vi "Do Failure Action.vi"(7 "Assert Data":T1, 8 "error in (no error)":errorcluster, 11 "Failure Action in":refnum<class "Failure Action.lvclass">) -> (0 "error out":errorcluster)   [LabVIEW 2016, in "AssertEngine.lvlib" / "Failure Action.lvclass"]
uses:
  Failure Action.lvclass
  Log Assert/Assert Data.ctl
  AssertEngine.lvlib
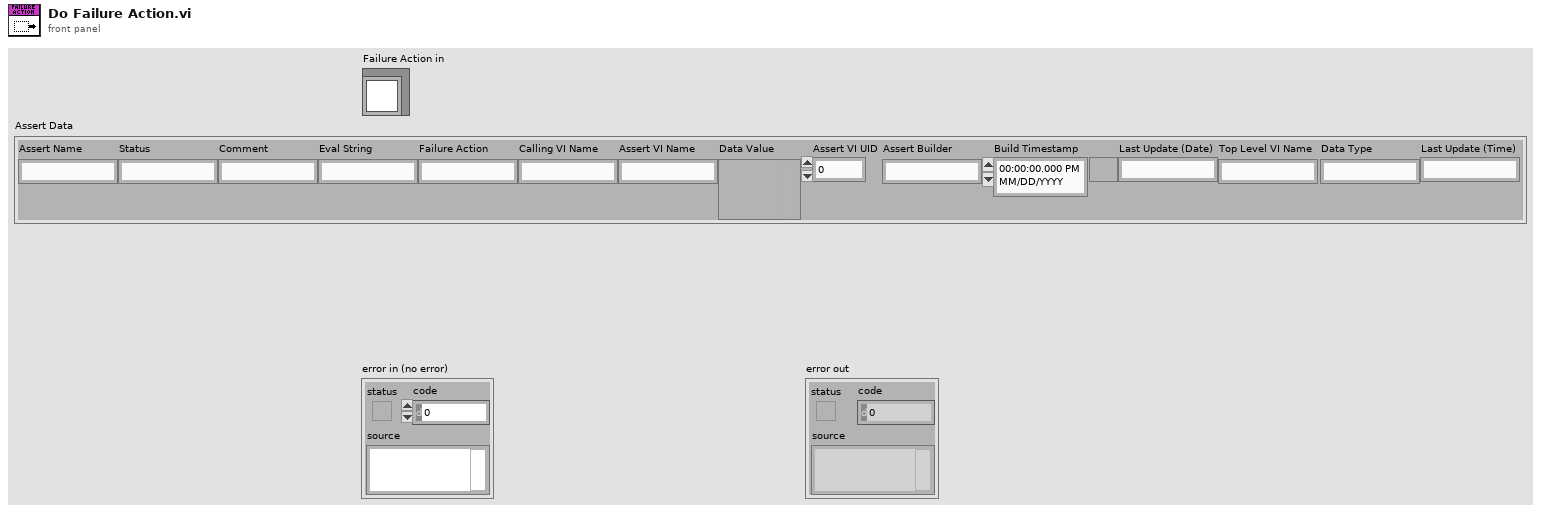
[diagram p1: front panel]
types:
  T1 = typedef "AssertEngine.lvlib/Assert Data.ctl" = cluster{"Assert Name":string, "Status":string, "Comment":string, "Eval String":string, "Failure Action":string, "Calling VI Name":string, "Assert VI Name":string, "Data Value":variant, "Assert VI UID":i32, "Assert Builder":string, "Build Timestamp":timestamp, "Last Update (Date)":string, "Top Level VI Name":string, "Data Type":string, "Last Update (Time)":string}
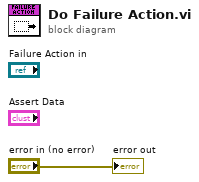
[diagram p0: block diagram]
diagram:
  "error out" <- "error in (no error)"
